vi "Set_RegData.vi"(8 "error in (no error)":errorcluster, 10 "data":T1, 11 "Class in":refnum<class "IB_RegData.lvclass">) -> (0 "error out":errorcluster, 3 "Class out":refnum<class "IB_RegData.lvclass">)   [LabVIEW 2020, in "IB_RegData.lvclass"]
uses:
  <vilib>/AppBuilder/IB_Classes/RegData/IB_RegData.lvclass
  <vilib>/AppBuilder/IB_Classes/RegData/IB_RegData.lvclass/IB_RegData.ctl
  <vilib>/AppBuilder/IB_Classes/RegData/IB_RegData.ctl
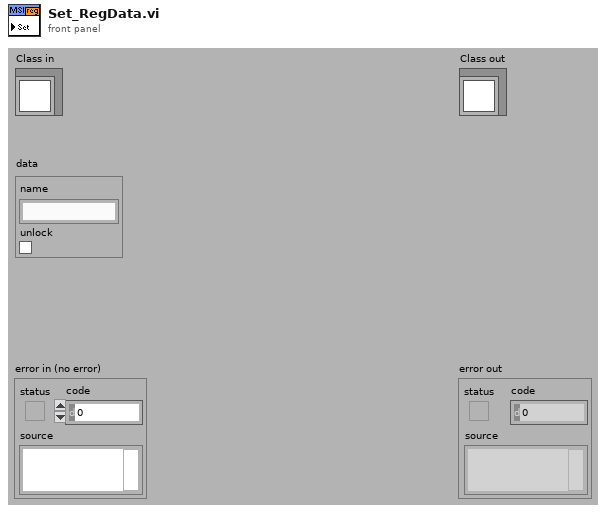
[diagram p1: front panel]
types:
  T1 = typedef "IB_RegData.ctl" = cluster{"name":string, "unlock":bool}
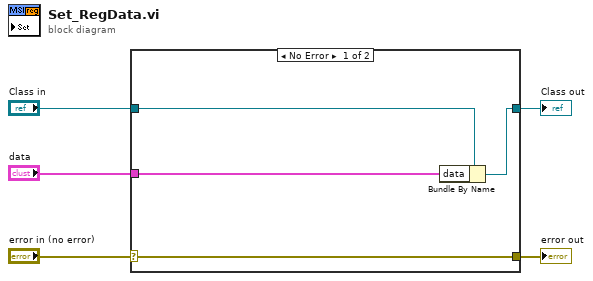
[diagram p0: block diagram]
diagram:
  n1 = case shown="No Error" "error in (no error)" {
    selector: "error in (no error)" -> [w9 w10]
    tunnel: [w9 w10] -> w4
    tunnel: [w7 w11] -> w2
    tunnel: "Class in" -> [w8 w11]
    tunnel: "data" -> [w6 _]
    frame No Error {
      n2 = Bundle By Name(cluster=w8, "data"=w6) -> (w7:refnum<class "IB_RegData.lvclass">)
    }
    frame Error {
    }
  }
  "error out" <- w4
  "Class out" <- w2
